vi "PID for Voltage.vi"(1 "ControlArray":T1(array[cluster])=[{"Name"="Volt_Direct", "PI Far->Close"=[], "FFinfo"={"FF_m"=0.0, "FF_b"=0.0}, "Limits"={"StepSize"=1e-05, "Max"=10.0, "Min"=0.0, "IndMin"=0.0}}, {"Name"="Volt_Flow", "PI Far->Close"=[], "FFinfo"={"FF_m"=0.0, "FF_b"=0.0}, "Limits"={"StepSize"=1e-05, "Max"=10.0, "Min"=0.0, "IndMin"=0.0}}, {"Name"="Volt_Speed", "PI Far->Close"=[], "FFinfo"={"FF_m"=0.0, "FF_b"=0.0}, "Limits"={"StepSize"=1e-05, "Max"=10.0, "Min"=0.0, "IndMin"=0.0}}, {"Name"="Pres_Direct", "PI Far->Close"=[], "FFinfo"={"FF_m"=0.0, "FF_b"=0.0}, "Limits"={"StepSize"=1e-05, "Max"=10.0, "Min"=0.0, "IndMin"=0.0}}, {"Name"="Pres_Flow", "PI Far->Close"=[], "FFinfo"={"FF_m"=0.0, "FF_b"=0.0}, "Limits"={"StepSize"=1e-05, "Max"=10.0, "Min"=0.0, "IndMin"=0.0}}, {"Name"="Pres_Speed", "PI Far->Close"=[], "FFinfo"={"FF_m"=0.0, "FF_b"=0.0}, "Limits"={"StepSize"=1e-05, "Max"=10.0, "Min"=0.0, "IndMin"=0.0}}, {"Name"="CMD_Direct", "PI Far->Close"=[], "FFinfo"={"FF_m"=0.0, "FF_b"=0.0}, "Limits"={"StepSize"=1e-05, "Max"=10.0, "Min"=0.0, "IndMin"=0.0}}, {"Name"="CMD_Flow", "PI Far->Close"=[], "FFinfo"={"FF_m"=0.0, "FF_b"=0.0}, "Limits"={"StepSize"=1e-05, "Max"=10.0, "Min"=0.0, "IndMin"=0.0}}, {"Name"="CMD_Speed", "PI Far->Close"=[], "FFinfo"={"FF_m"=0.0, "FF_b"=0.0}, "Limits"={"StepSize"=1e-05, "Max"=10.0, "Min"=0.0, "IndMin"=0.0}}], 3 "Feedback":dbl[](array[numeric]), 5 "CommandCluster":T2, 9 "VandPLimits":dbl[](array[numeric]), 13 "Controller?":bool) -> (4 "PIdata":dbl[](array[numeric]), 8 "Output":dbl)   [LabVIEW 2013]
uses:
  TypeDef/Command Cluster.ctl
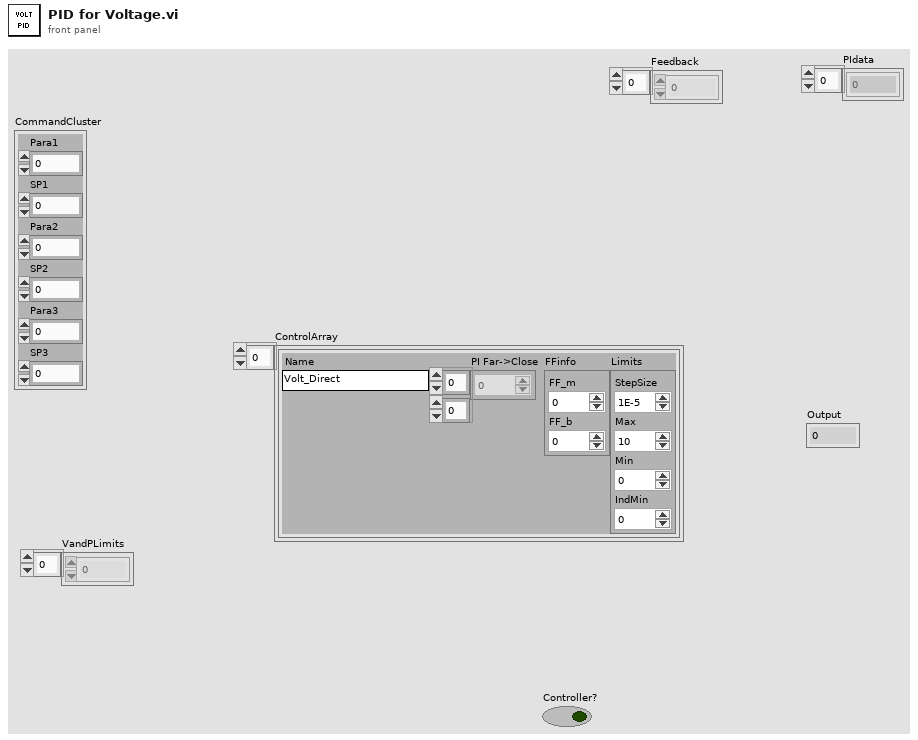
[diagram p1: front panel]
types:
  T1 = cluster{"Name":string, "PI Far->Close":dbl[][], "FFinfo":cluster{"FF_m":dbl, "FF_b":dbl}, "Limits":cluster{"StepSize":dbl, "Max":dbl, "Min":dbl, "IndMin":dbl}}[]
  T2 = typedef "Command Cluster.ctl" = cluster{"Para1":i32, "SP1":dbl, "Para2":i32, "SP2":dbl, "Para3":i32, "SP3":dbl}
  T3 = cluster{"Name":string, "PI Far->Close":dbl[][], "FFinfo":cluster{"FF_m":dbl, "FF_b":dbl}, "Limits":cluster{"StepSize":dbl, "Max":dbl, "Min":dbl, "IndMin":dbl}}
  T4 = cluster{"StepSize":dbl, "Max":dbl, "Min":dbl, "IndMin":dbl}
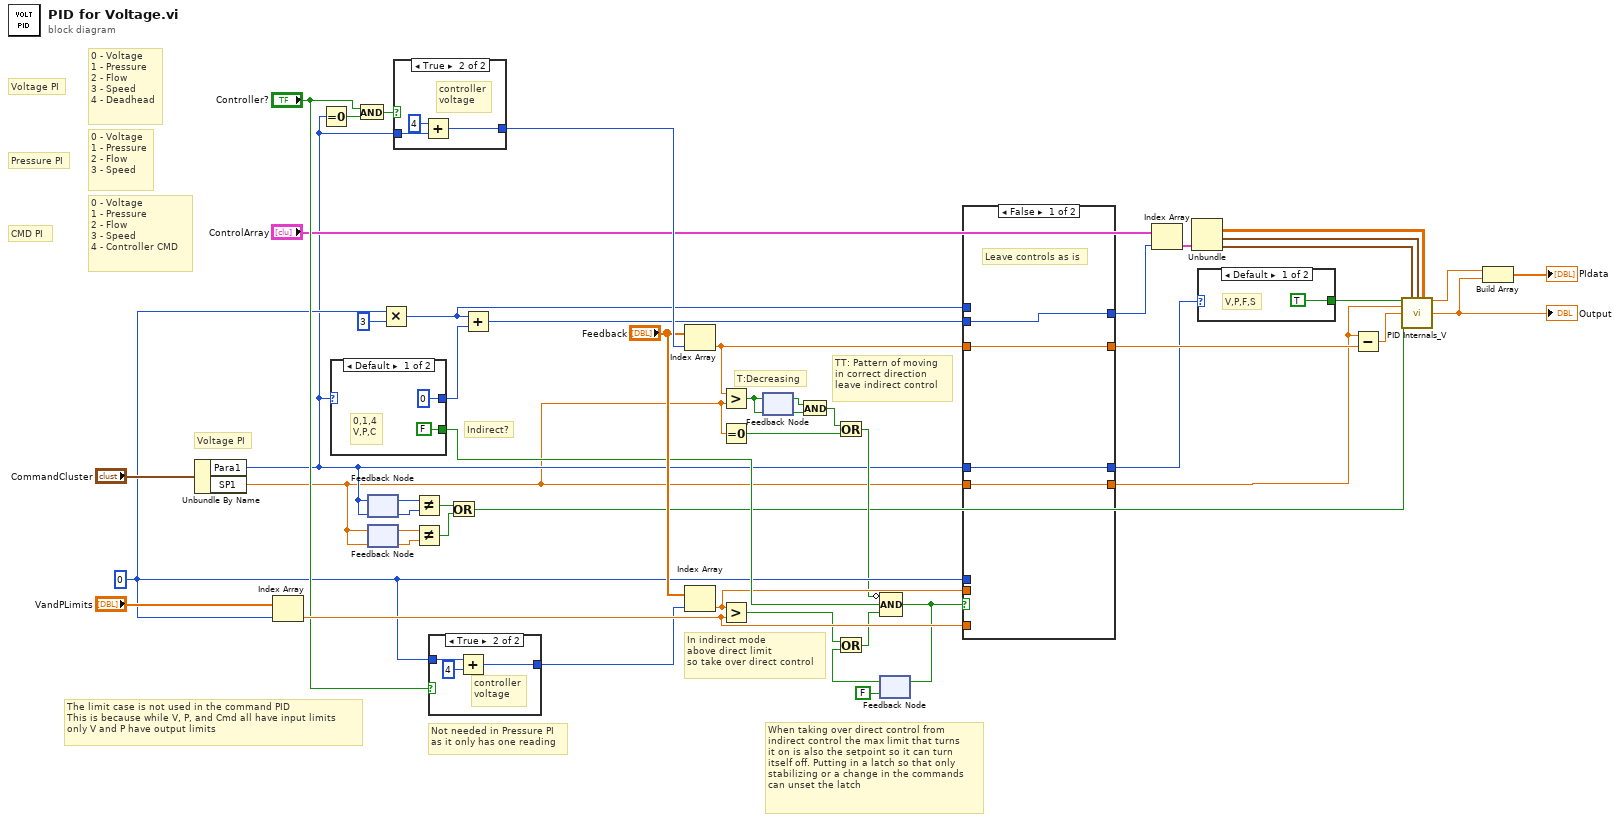
[diagram p0: block diagram]
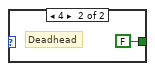
[diagram p2: hidden frame]
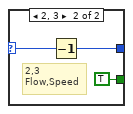
[diagram p6: hidden frame]
diagram:
  w28 = 0 ("CtrlIndex")
  # "Voltage PI"
  # "When taking over direct control from\nindirect control the max limit that turns\nit on is also the setpoint so it can turn\nitself off. Putting in a latch so that only\nstabilizing or a change in the commands\ncan unset the latch"
  # "Not needed in Pressure PI\nas it only has one reading"
  # "TT: Pattern of moving\nin correct direction\nleave indirect control"
  # "In indirect mode\nabove direct limit\nso take over direct control"
  # "T:Decreasing"
  # "The limit case is not used in the command PID\nThis is because while V, P, and Cmd all have input limits\nonly V and P have output limits"
  # "Indirect?"
  # "CMD PI"
  # "Pressure PI"
  # "Voltage PI"
  # "0 - Voltage\n1 - Pressure\n2 - Flow\n3 - Speed\n4 - Controller CMD"
  # "0 - Voltage\n1 - Pressure\n2 - Flow\n3 - Speed"
  # "0 - Voltage\n1 - Pressure\n2 - Flow\n3 - Speed\n4 - Deadhead"
  n1 = Unbundle By Name("CommandCluster") -> ("Para1"=w6:i32, "SP1"=w4:dbl)
  n2 = Index Array(array="VandPLimits", index=w28) -> (element=w31:dbl)
  n3 = Equal To 0?(x=w6) -> (x = 0?=w42:bool)
  n4 = case shown="Default" w6 {
    selector: w6 -> [_ w53]
    tunnel: [0 w52] -> w44
    tunnel: [FALSE TRUE] -> w36
    frame Default {
      # "0,1,4\nV,P,C"
    }
    frame 2, 3 {
      # "2,3\nFlow,Speed"
      n5 = Decrement(x=w53) -> (x-1=w52:i32)
    }
  }
  n6 = And(x="Controller?", y=w42) -> (x .and. y?=w43:bool)
  n7 = feedback #1(w6) -> (w7:i32)
  n8 = feedback-in #1(w6) -> ()
  n9 = feedback #2(w4) -> (w5:dbl)
  n10 = feedback-in #2(w4) -> ()
  n11 = Multiply(x=w28, y=3) -> (x*y=w30:i32)
  n12 = case shown="True" w43 {
    tunnel: w6 -> [w54 w57]
    tunnel: [w54 w55] -> w40
    frame False {
      # "pump\nvoltage"
    }
    frame True {
      # "controller\nvoltage"
      n13 = Add(x=4, y=w57) -> (x+y=w55:i32)
    }
  }
  n14 = Not Equal?(x=w7, y=w6) -> (x != y?=w2:bool)
  n15 = Not Equal?(x=w5, y=w4) -> (x != y?=w3:bool)
  n16 = case shown="True" "Controller?" {
    tunnel: [w58 w61] -> w27
    tunnel: w28 -> [w58 w60]
    frame False {
      # "pump\nvoltage"
    }
    frame True {
      # "controller\nvoltage"
      n17 = Add(x=w60, y=4) -> (x+y=w61:i32)
    }
  }
  n18 = Or(x=w2, y=w3) -> (x .or. y?=w1:bool)
  n19 = Add(x=w30, y=w44) -> (x+y=w33:i32)
  n20 = Index Array(array="Feedback", index=w40) -> (element=w35:dbl)
  n21 = Index Array(array="Feedback", index=w27) -> (element=w32:dbl)
  n22 = Greater?(x=w35, y=w4) -> (0:w37:bool)
  n23 = Equal To 0?(x=w4) -> (x = 0?=w26:bool)
  n24 = Greater?(x=w32, y=w31) -> (0:w20:bool)
  n25 = feedback #3(w37) -> (w38:bool)
  n26 = feedback-in #3(w37) -> ()
  n27 = And(x=w38, y=w37) -> (x .and. y?=w25:bool)
  n28 = Or(x=w25, y=w26) -> (x .or. y?=w24:bool)
  n29 = feedback #4(FALSE) -> (w21:bool)
  n30 = Or(x=w20, y=w21) -> (x .or. y?=w19:bool)
  n31 = Compound Arithmetic op=AND(invert w24, w36, w19) -> (w23:bool)
  n32 = feedback-in #4(w23) -> ()
  n33 = case shown="False" w23 {
    tunnel: w6 -> [w65 _]
    tunnel: w4 -> [w64 _]
    tunnel: [w65 w68] -> w18
    tunnel: [w64 w69] -> w17
    tunnel: w35 -> [w63 _]
    tunnel: [w63 w67] -> w34
    tunnel: w33 -> [w62 _]
    tunnel: [w62 w66] -> w12
    tunnel: w32 -> [_ w67]
    tunnel: w31 -> [_ w69]
    tunnel: w28 -> [_ w68]
    tunnel: w30 -> [_ w66]
    frame False {
      # "Leave controls as is"
    }
    frame True {
      # "Change from indirect\nto direct control due\nto over limit"
    }
  }
  n34 = Index Array(array="ControlArray", index=w12) -> (element=w11:T3)
  n35 = Unbundle(w11) -> ("PI Far->Close"=w10:dbl[][], "FFinfo"=w9:cluster{"FF_m":dbl, "FF_b":dbl}, "Limits"=w8:T4)  [unwired: 1 out]
  n36 = case shown="Default" w18 {
    tunnel: [TRUE FALSE] -> w16
    frame Default {
      # "V,P,F,S"
    }
    frame 4 {
      # "Deadhead"
    }
  }
  n37 = Subtract(x=w17, y=w34) -> (x-y=w15:dbl)
  n38 = call "PID Internals_V.vi"("Run PI?"=w16, "LimitCluster"=w8, "FFcluster"=w9, "PI Far->Close"=w10, "SP"=w17, "Error"=w15, "CMDchanged"=w1) -> ("SlewIndex"=w14:dbl, "Output"=w47:dbl)  [unwired: 7 in]
  "Output" <- w47
  n39 = Build Array(w14, w47) -> (→"PIdata":dbl[])
